vi "RT-Tanh.vi"(1 "x":dbl) -> (0 "tanh":dbl)   [LabVIEW 2020]
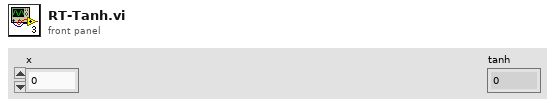
[diagram p1: front panel]
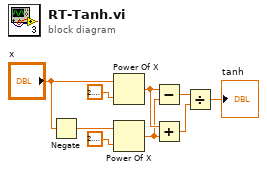
[diagram p0: block diagram]
diagram:
  n1 = Negate(x="x") -> (-x=w7:dbl)
  n2 = Power Of X(1:2.718281828459045, 2:"x") -> (0:w5:dbl)
  n3 = Power Of X(1:2.718281828459045, 2:w7) -> (0:w4:dbl)
  n4 = Subtract(x=w5, y=w4) -> (x-y=w3:dbl)
  n5 = Add(x=w5, y=w4) -> (x+y=w2:dbl)
  n6 = Divide(x=w3, y=w2) -> (x/y=→"tanh":dbl)
